vi "Field Draw Target.vi"(4 "Lado":enum16{"Esquerdo", "Direito"}(ring) caption="Enum", 6 "Draw Targets?":T2, 7 "Dest":T1, 8 "picture in":picture, 9 "Offset":T8, 10 "Scale mm/pixel":dbl, 11 "Robot":T4={"id"=0, "function"=enum."Attacker", "x"=0.0, "y"=0.0, "orientation"=0.0, "v_tangent"=0.0, "v_normal"=0.0, "v_ang"=0.0, "kick_x"=0.0, "kick_z"=0.0, "dribble"=FALSE, "Timestamp"=timestamp(0 s since 1904-01-01), "estimatives"={"est_v_tangent"=0.0, "est_v_normal"=0.0, "est_vx"=0.0, "est_vy"=0.0, "Pos Robot Est"=[]}, "dest_x_kick"=0.0, "dest_y_kick"=0.0, "Gap Coord"=[], "States"=enum."GoToTangent", "Path "=[], "Path  Smooth"=[], "Dest"=[]}) -> (0 "picture out":picture)   [LabVIEW 2017]
uses:
  <vilib>/Utility/miscctls.llb/LVBoundsTypeDef.ctl
  Core/AI Robot.ctl
  Intel/Functions Enum.ctl
  Intel/AttackerStates.ctl
  Path Planning/RRT/PathDests.ctl
  Path Planning/RRT/PathDest.ctl
  <vilib>/Analysis/coordinate.llb/Angle Range (Degree).ctl
  DrawTargets.ctl
  <vilib>/Analysis/coordinate.llb/2D Cartesian Coordinate Rotation (Scalar).vi
  <vilib>/Analysis/NI_AAL_Angle.lvlib
  <vilib>/Analysis/NI_AALPro.lvlib
  <vilib>/Analysis/coordinate.llb/Wrap Angle (scalar).vi
panel:
  in  "angle range":T3=1
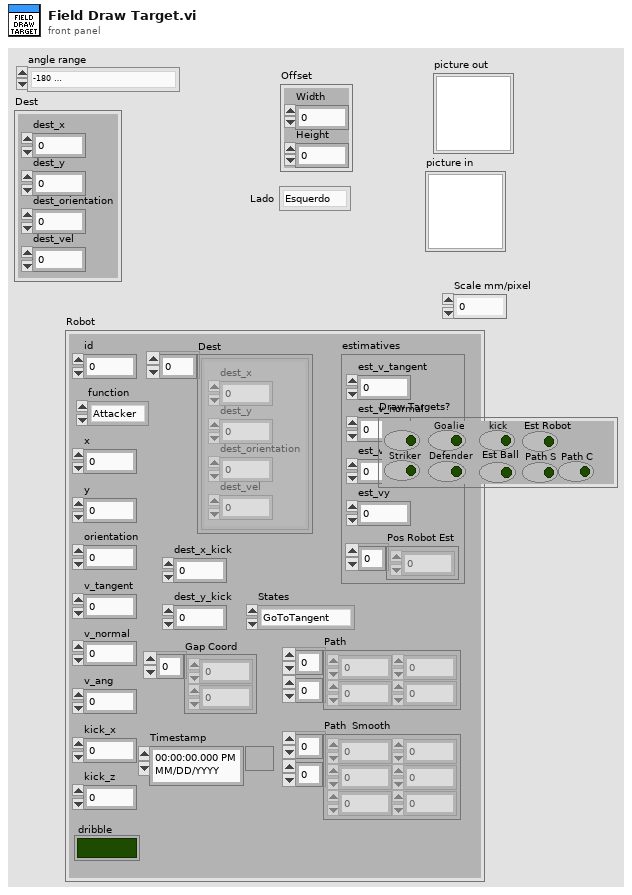
[diagram p1: front panel]
types:
  T1 = typedef "PathDest.ctl" = cluster{"dest_x":dbl, "dest_y":dbl, "dest_orientation":dbl, "dest_vel":dbl}
  T2 = typedef "DrawTargets.ctl" = cluster{"Attacker":bool, "Striker":bool, "Goalie":bool, "Defender":bool, "kick":bool, "Est Ball":bool, "Est Robot":bool, "Path S":bool, "Path C":bool}
  T3 = typedef "NI_AAL_Angle.lvlib/Angle Range (Degree).ctl" = u16
  T4 = typedef "AI Robot.ctl" = cluster{"id":u32, "function":T5, "x":dbl, "y":dbl, "orientation":dbl, "v_tangent":dbl, "v_normal":dbl, "v_ang":dbl, "kick_x":dbl, "kick_z":dbl, "dribble":bool, "Timestamp":timestamp, "estimatives":cluster{"est_v_tangent":dbl, "est_v_normal":dbl, "est_vx":dbl, "est_vy":dbl, "Pos Robot Est":dbl[]}, "dest_x_kick":dbl, "dest_y_kick":dbl, "Gap Coord":dbl[], "States":T6, "Path ":dbl[][], "Path  Smooth":dbl[][], "Dest":T7}
  T5 = typedef "Functions Enum.ctl" = enum16{"Attacker", "Goalie", "Defender", "Striker", "Goto 0", "Dummy", "Kicker", "ZigZag"}
  T6 = typedef "AttackerStates.ctl" = enum16{"Pass", "GoToTangent", "BallGetting", "GoToKick", ""}
  T7 = typedef "PathDests.ctl" = T1[]
  T8 = typedef "LVBoundsTypeDef.ctl" = cluster{"Width":u32, "Height":u32}
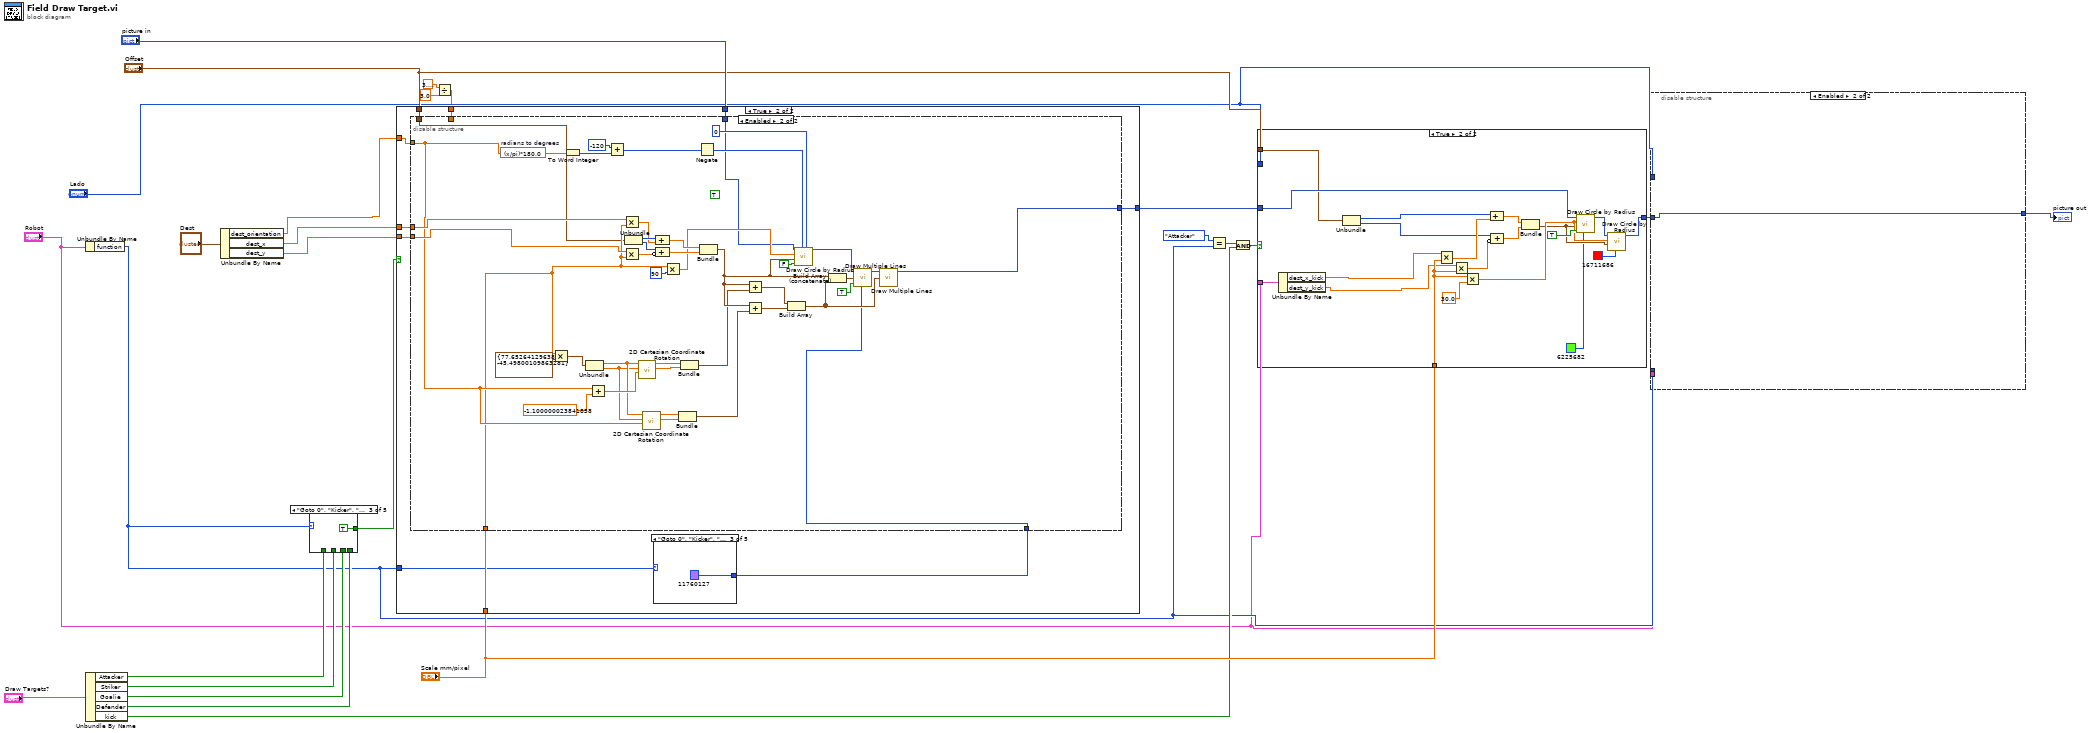
[diagram p0: block diagram]
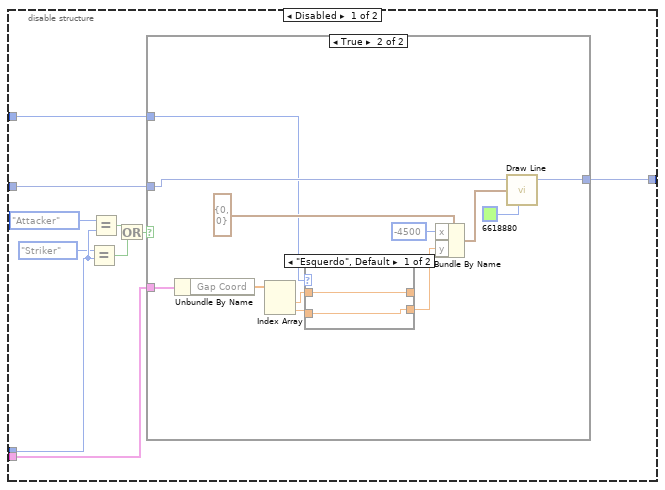
[diagram p2: hidden frame]
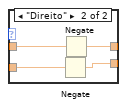
[diagram p4: hidden frame]
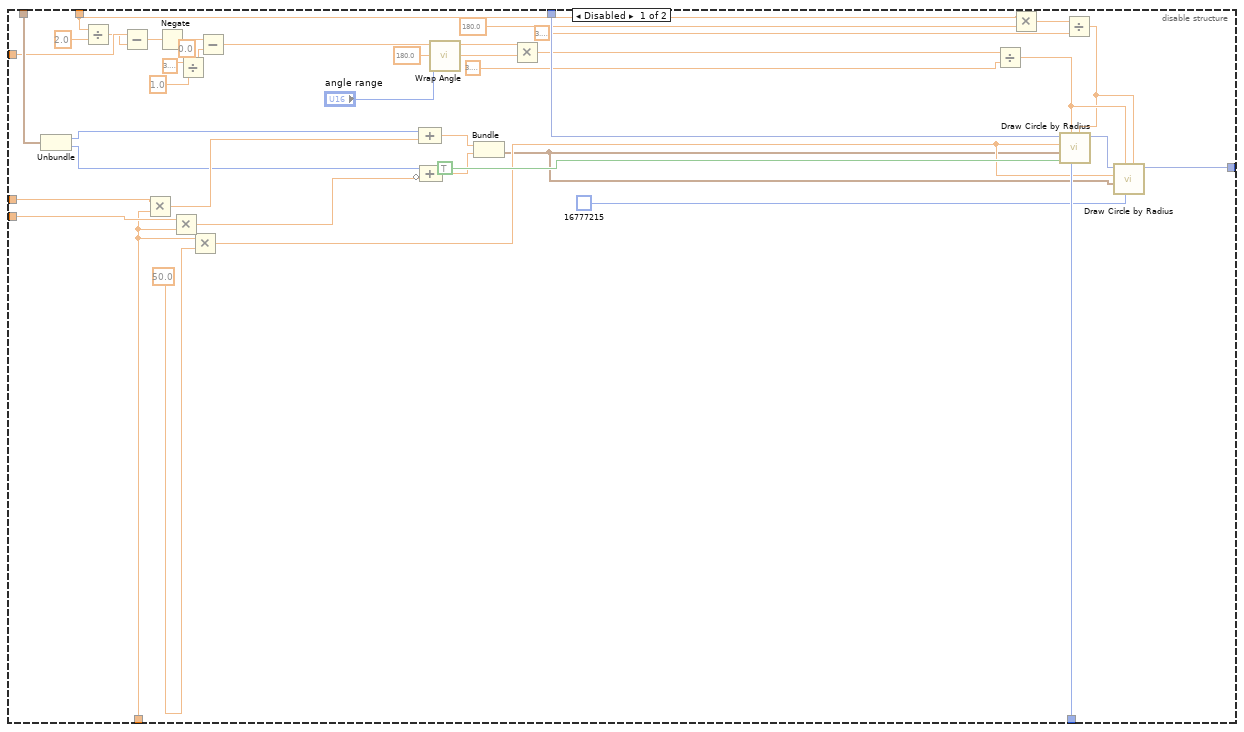
[diagram p10: hidden frame]
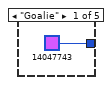
[diagram p11: hidden frame]
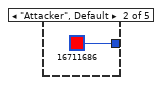
[diagram p12: hidden frame]
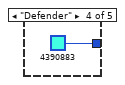
[diagram p13: hidden frame]
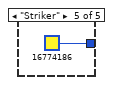
[diagram p14: hidden frame]
diagram:
  n1 = Unbundle By Name("Robot") -> ("function"=w12:T5)
  n2 = Unbundle By Name("Draw Targets?") -> ("Attacker"=w19:bool, "Striker"=w20:bool, "Goalie"=w18:bool, "Defender"=w21:bool, "kick"=w16:bool)
  n3 = Unbundle By Name("Dest") -> ("dest_orientation"=w8:dbl, "dest_x"=w3:dbl, "dest_y"=w2:dbl)
  n4 = case shown="\"Goto 0\", \"Kicker\", \"ZigZag\"" w12 {
    tunnel: [w27 w28 TRUE ("Draw Target Striker?") w30 w31] -> w22
    tunnel: w21 -> [_ _ _ w30 _]
    tunnel: w20 -> [_ _ _ _ w31]
    tunnel: w19 -> [w27 _ _ _ _]
    tunnel: w18 -> [_ w28 _ _ _]
    frame "Attacker", Default {
    }
    frame "Goalie" {
    }
    frame "Goto 0", "Kicker", "ZigZag" {
    }
    frame "Defender" {
    }
    frame "Striker" {
    }
  }
  n5 = Divide(x=3.141592653589793, y=3.0) -> (x/y=w7:dbl)
  n6 = case shown="True" w22 {
    tunnel: w2 -> [_ w41]
    tunnel: w3 -> [_ w40]
    tunnel: "picture in" -> [w32 w39]
    tunnel: [w32 w38] -> w25
    tunnel: "Offset" -> [_ w37]
    tunnel: "Scale mm/pixel" -> [_ w36]
    tunnel: w12 -> [_ w35]
    tunnel: w8 -> [_ w34]
    tunnel: w7 -> [_ w33]
    frame False {
    }
    frame True {
      n7 = case shown="\"Goto 0\", \"Kicker\", \"ZigZag\"" w35 {
        tunnel: [u32 14047743 ("color(black)") u32 16711686 ("color(black)") u32 11760127 ("color(black)") u32 4390883 ("color(black)") u32 16774186 ("color(black)")] -> w42
        frame "Goalie" {
        }
        frame "Attacker", Default {
        }
        frame "Goto 0", "Kicker", "ZigZag" {
        }
        frame "Defender" {
        }
        frame "Striker" {
        }
      }
      n8 = disable-structure shown="Enabled" {
        disable-tunnel: w42 -> [w80 w83]
        disable-tunnel: w41 -> [w78 w88]
        disable-tunnel: w40 -> [w77 w89]
        disable-tunnel: w39 -> [w70 w86]
        disable-tunnel: [w66 w85] -> w38
        disable-tunnel: w37 -> [w65 w82]
        disable-tunnel: w36 -> [w64 w84]
        disable-tunnel: w34 -> [w55 w87]
        disable-tunnel: w33 -> [w52 _]
        frame Disabled {
          (unwired) 0.0 ("y")
          n9 = Unbundle(w65) -> ("Width"=w76:u32, "Height"=w73:u32)
          n10 = Divide(x=w52, y=2.0) -> (x/y=w54:dbl)
          n11 = Subtract(x=w55, y=w54) -> (x-y=w61:dbl)
          n12 = Multiply(x=w77, y=w64) -> (x*y=w75:dbl)
          n13 = Negate(x=w61) -> (-x=w60:dbl)
          n14 = Multiply(x=w78, y=w64) -> (x*y=w72:dbl)
          n15 = Divide(x=3.141592653589793, y=1.0) -> (x/y=w43:dbl)
          n16 = Multiply(x=w64, y=sgl 50.0 ("radius")) -> (x*y=w68:dbl)
          n17 = Subtract(x=w60, y=w43) -> (x-y=w56:dbl)
          n18 = Compound Arithmetic op=ADD(w76, w75) -> (w74:dbl)
          n19 = Compound Arithmetic op=ADD(w73, invert w72) -> (w71:dbl)
          n20 = call-poly <vilib>:"Wrap Angle.vi"("angle range"="angle range", "angle in"=w56) -> ("angle out"=w53:dbl)  [unwired: 8 in, 1 out]
          n21 = Bundle(w74, w71) -> (w67:cluster{dbl, dbl})  [unwired: 1 in]
          n22 = Multiply(x=w53, y=180.0) -> (x*y=w50:dbl)
          n23 = Divide(x=w50, y=3.141592653589793) -> (x/y=w45:dbl)
          n24 = Multiply(x=w52, y=180.0) -> (x*y=w51:dbl)
          n25 = Divide(x=w51, y=3.141592653589793) -> (x/y=w44:dbl)
          n26 = call <vilib>:"Draw Circle by Radius.vi"("arc size(360)"=w44, "color(black)"=w80, "start angle(0)"=w45, "fill?(F)"=TRUE, "pixel center"=w67, "radius"=w68, "picture"=w70) -> ("new picture"=w69:picture)  [unwired: 4 in]
          n27 = call <vilib>:"Draw Circle by Radius.vi"("arc size(360)"=w44, "color(black)"=u32 16777215, "start angle(0)"=w45, "pixel center"=w67, "radius"=w68, "picture"=w69) -> ("new picture"=w66:picture)  [unwired: 5 in]
        }
        frame Enabled {
          (unwired) TRUE ("fill?(F)")
          n28 = expression code="(x/pi)*180.0" "radians to degrees"(w87) -> (w116:dbl)
          n29 = Multiply(x=w84, y=cluster{sgl, sgl} {77.65264, -45.498} ("appended array")) -> (x*y=w95:cluster{dbl, dbl})
          n30 = To Word Integer(number=w116) -> (16bit integer=w115:i16)
          n31 = Unbundle(w95) -> (w100:dbl, w99:dbl)
          n32 = Add(x=w87, y=sgl -1.1 ("theta")) -> (x+y=w101:dbl)
          n33 = Add(x=i16 -120, y=w115) -> (x+y=w114:i16)
          n34 = Multiply(x=w89, y=w84) -> (x*y=w122:dbl)
          n35 = Multiply(x=w88, y=w84) -> (x*y=w119:dbl)
          n36 = Unbundle(w82) -> ("Width"=w123:u32, "Height"=w120:u32)
          n37 = call-poly <vilib>:"2D Cartesian Coordinate Rotation.vi"("theta"=w101, "y"=w99, "x"=w100) -> ("y out"=w103:dbl, "x out"=w104:dbl)  [unwired: 6 in, 1 out]
          n38 = call-poly <vilib>:"2D Cartesian Coordinate Rotation.vi"("theta"=w87, "y"=w99, "x"=w100) -> ("y out"=w97:dbl, "x out"=w98:dbl)  [unwired: 6 in, 1 out]
          n39 = Compound Arithmetic op=ADD(w123, w122) -> (w121:dbl)
          n40 = Compound Arithmetic op=ADD(w120, invert w119) -> (w118:dbl)
          n41 = Multiply(x=w84, y=i16 90 ("radius")) -> (x*y=w110:dbl)
          n42 = Bundle("x out"=w98, "y out"=w97) -> (w94:cluster{"x out":dbl, "y out":dbl})  [unwired: 1 in]
          n43 = Bundle("x out"=w104, "y out"=w103) -> (w93:cluster{"x out":dbl, "y out":dbl})  [unwired: 1 in]
          n44 = Negate(x=w114) -> (-x=w112:i16)
          n45 = Bundle(w121, w118) -> (w109:cluster{dbl, dbl})  [unwired: 1 in]
          n46 = Add(x=w109, y=w93) -> (x+y=w91:cluster{dbl, dbl})
          n47 = Add(x=w109, y=w94) -> (x+y=w92:cluster{dbl, dbl})
          n48 = Build Array(w91, w92) -> (w108:cluster{dbl, dbl}[])
          n49 = call <vilib>:"Draw Circle by Radius.vi"("arc size(360)"=i16 0, "start angle(0)"=w112, "fill?(F)"=FALSE, "pixel center"=w109, "radius"=w110, "picture"=w86) -> ("new picture"=w90:picture)  [unwired: 5 in]
          n50 = Build Array (concatenate)(w109, w108) -> (w106:cluster{dbl, dbl}[])
          n51 = call <vilib>:"Draw Multiple Lines.vi"("picture"=w90, "line endpoints"=w106, "fill?(F)"=TRUE, "color(black)"=w83) -> ("new picture"=w107:picture)  [unwired: 5 in]
          n52 = call <vilib>:"Draw Multiple Lines.vi"("picture"=w107, "line endpoints"=w108) -> ("new picture"=w85:picture)  [unwired: 7 in]
        }
      }
    }
  }
  n53 = Equal?(x=Functions_Enum."Attacker" ("y"), y=w12) -> (x = y?=w15:bool)
  n54 = And(x=w15, y=w16) -> (x .and. y?=w17:bool)
  n55 = case shown="True" w17 {
    tunnel: w25 -> [w130 w139]
    tunnel: [w130 w138] -> w13
    tunnel: "Robot" -> [_ w137]
    tunnel: "Offset" -> [_ w136]
    tunnel: "Scale mm/pixel" -> [_ w135]
    tunnel: "Lado" -> [_ _]
    frame False {
    }
    frame True {
      n56 = Unbundle By Name(w137) -> ("dest_x_kick"=w132:dbl, "dest_y_kick"=w131:dbl)
      n57 = Unbundle(w136) -> ("Width"=w148:u32, "Height"=w145:u32)
      n58 = Multiply(x=w132, y=w135) -> (x*y=w147:dbl)
      n59 = Multiply(x=w131, y=w135) -> (x*y=w144:dbl)
      n60 = Multiply(x=w135, y=sgl 30.0 ("radius")) -> (x*y=w141:dbl)
      n61 = Compound Arithmetic op=ADD(w148, w147) -> (w146:dbl)
      n62 = Compound Arithmetic op=ADD(w145, invert w144) -> (w143:dbl)
      n63 = Bundle(w146, w143) -> (w140:cluster{dbl, dbl})  [unwired: 1 in]
      n64 = call <vilib>:"Draw Circle by Radius.vi"("color(black)"=u32 6225682, "fill?(F)"=TRUE, "pixel center"=w140, "radius"=w141, "picture"=w139) -> ("new picture"=w142:picture)  [unwired: 6 in]
      n65 = call <vilib>:"Draw Circle by Radius.vi"("color(black)"=u32 16711686, "pixel center"=w140, "radius"=w141, "picture"=w142) -> ("new picture"=w138:picture)  [unwired: 7 in]
    }
  }
  n66 = disable-structure shown="Enabled" {
    disable-tunnel: w13 -> [w160 w180]
    disable-tunnel: w12 -> [w159 _]
    disable-tunnel: [w153 w180] -> w11
    disable-tunnel: "Robot" -> [w152 _]
    disable-tunnel: "Lado" -> [w151 _]
    frame Disabled {
      n67 = Equal?(x=Functions_Enum."Striker", y=w159) -> (x = y?=w154:bool)
      n68 = Equal?(x=Functions_Enum."Attacker", y=w159) -> (x = y?=w155:bool)
      n69 = Or(x=w155, y=w154) -> (x .or. y?=w156:bool)
      n70 = case shown="True" w156 {
        tunnel: w160 -> [w161 w169]
        tunnel: [w161 w170] -> w153
        tunnel: w152 -> [_ w173]
        tunnel: w151 -> [_ w163]
        frame False {
        }
        frame True {
          n71 = Unbundle By Name(w173) -> ("Gap Coord"=w171:dbl[])
          n72 = Index Array(array=w171) -> (element #1=w166:dbl, element #2=w165:dbl)  [unwired: 2 in]
          n73 = case shown="\"Esquerdo\", Default" w163 {
            tunnel: [w175 w179] -> _
            tunnel: w166 -> [w175 w177]
            tunnel: [w174 w178] -> w164
            tunnel: w165 -> [w174 w176]
            frame "Esquerdo", Default {
            }
            frame "Direito" {
              n74 = Negate(x=w176) -> (-x=w178:dbl)
              n75 = Negate(x=w177) -> (-x=w179:dbl)
            }
          }
          n76 = Bundle By Name(cluster=cluster{"x":i16, "y":i16} {"x"=0, "y"=0} ("end point"), "x"=i16 -4500, "y"=w164) -> (w168:cluster{"x":i16, "y":i16})
          n77 = call <vilib>:"Draw Line.vi"("picture"=w169, "end point"=w168, "color(black)"=u32 6618880) -> ("new picture"=w170:picture)  [unwired: 6 in]
        }
      }
    }
    frame Enabled {
    }
  }
  "picture out" <- w11
